vi "Global - Obstacles.vi"(7 "mode":enum16{"Initialize", "Read", "Write"}(ring), 8 "error in (no error)":errorcluster, 10 "obstacles in":cluster{dbl, dbl}[][](array[cluster])) -> (0 "error out":errorcluster, 1 "failed?":bool, 2 "obstacles out":cluster{dbl, dbl}[][](array[cluster]))   [LabVIEW 2011]
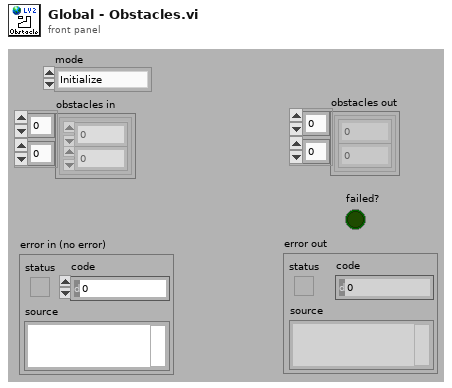
[diagram p1: front panel]
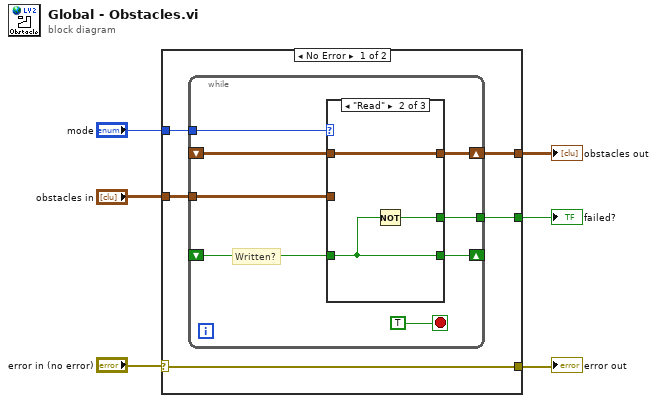
[diagram p0: block diagram]
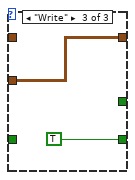
[diagram p3: hidden frame]
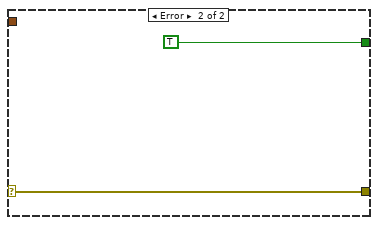
[diagram p4: hidden frame]
diagram:
  n1 = case shown="No Error" "error in (no error)" {
    selector: "error in (no error)" -> [w7 w26]
    tunnel: [w7 w26] -> w5
    tunnel: "mode" -> [w11 _]
    tunnel: "obstacles in" -> [w10 _]
    tunnel: [w9 _] -> w2
    tunnel: [w8 TRUE] -> w1
    frame No Error {
      n2 = while {
        shift-right: [w16] -> w9
        shift-left: _ -> [w13]
        shift-right: [w17] -> _
        shift-left: _ -> [w14]
        tunnel: w11 -> [w18]
        tunnel: w10 -> [w15]
        tunnel: [w12] -> w8
        stop <- TRUE stop-if-true
        # "Written?"
        n3 = case shown="\"Read\"" w18 {
          tunnel: [_ w21 TRUE] -> w17
          tunnel: [_ w22 w23] -> w16
          tunnel: w15 -> [_ _ w23]
          tunnel: w14 -> [_ w21 _]
          tunnel: w13 -> [_ w22 _]
          tunnel: [_ w20 _] -> w12
          frame "Initialize" {
          }
          frame "Read" {
            n4 = Not(x=w21) -> (.not. x?=w20:bool)
          }
          frame "Write" {
          }
        }
      }
    }
    frame Error {
    }
  }
  "error out" <- w5
  "obstacles out" <- w2
  "failed?" <- w1
